vi "Target Check Safety Limits.vi"(11 "Sensors":T1) -> (3 "Limits Tripped":bool)   [LabVIEW 2018]
uses:
  Sensor Data.ctl
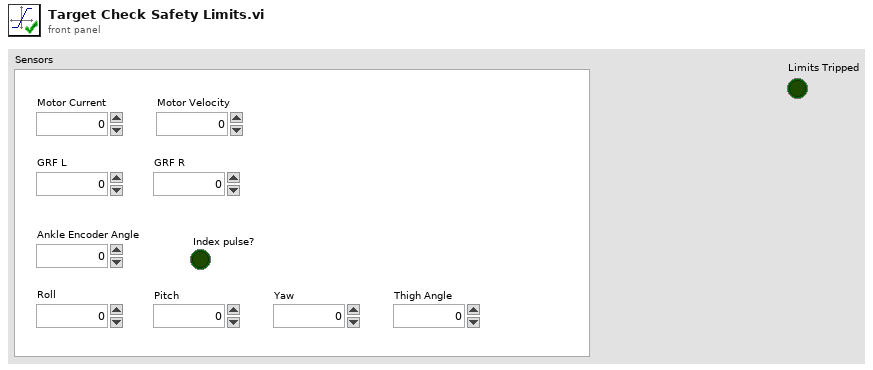
[diagram p1: front panel]
types:
  T1 = typedef "Sensor Data.ctl" = cluster{"Motor Current":dbl, "Motor Velocity":dbl, "Ankle Encoder Angle":dbl, "GRF L":dbl, "GRF R":dbl, "Index pulse?":bool, "Roll":dbl, "Pitch":dbl, "Yaw":dbl, "Thigh Angle":dbl}
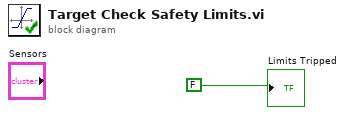
[diagram p0: block diagram]
diagram:
  "Limits Tripped" <- FALSE
